vi "Configure Process Value.vi"(6 "Sensor Break Type (0: Off)":u8(ring) items=["Off", "Low", "High"], 7 "Unit Address (1)":u8=1, 8 "error in (no error)":errorcluster, 9 "Filter Time Constant (0)":u16, 10 "PV Offset (0)":i32, 11 "VISA resource name":refnum<visa-resource-name>) -> (0 "error out":errorcluster, 3 "VISA resource name out":refnum<visa-resource-name>)   [LabVIEW 2014, in "Eurotherm 35xx Series.lvlib"]
doc: "This VI configure process variable parameters."
uses:
  <instrlib>/Eurotherm 35xx Series/Eurotherm 35xx Series.lvlib
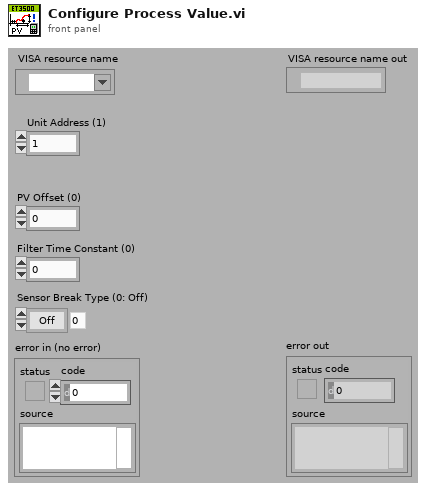
[diagram p1: front panel]
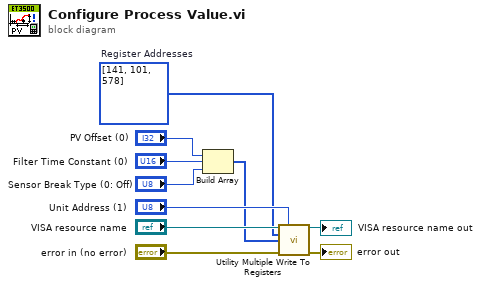
[diagram p0: block diagram]
diagram:
  w5 = i32[] [141, 101, 578]  # Register Addresses
  n1 = Build Array("PV Offset (0)", "Filter Time Constant (0)", "Sensor Break Type (0: Off)") -> (w4:i32[])
  n2 = call <instrlib>:"Utility Multiple Write To Registers.vi"("VISA resource name"="VISA resource name", "Unit Address (1)"="Unit Address (1)", "Registers Addresses (0)"=w5, "Data (0)"=w4, "error in (no error)"="error in (no error)") -> ("VISA resource name out"=→"VISA resource name out":refnum<visa-resource-name>, "error out"=→"error out":errorcluster)  [unwired: 9 in]
